vi "WindowArrayV0.42.vi"(0 "Searching center":dbl format="%.2f", 2 "X-axis":dbl[](array[numeric]) format="%.2f", 3 "The Data":dbl[](array[numeric]) format="%.2f", 5 "Window Width (point)":i32=80) -> (1 "scale":dbl format="%.2f", 4 "starting point":dbl format="%.2f", 6 "Closest peak position":dbl format="%.2f", 7 "X-Axis Subset":dbl[](array[numeric]) format="%.2f", 8 "Data Subset":dbl[](array[numeric]) format="%.2f")   [LabVIEW 2024]
doc: "Truncate the data around a peak. Normalize X-Axis so I can use the spline VI, and you can retrive the original X-Axis with *scale+StartingPoint."
uses:
  <vilib>/Analysis/NI_AALPro.lvlib
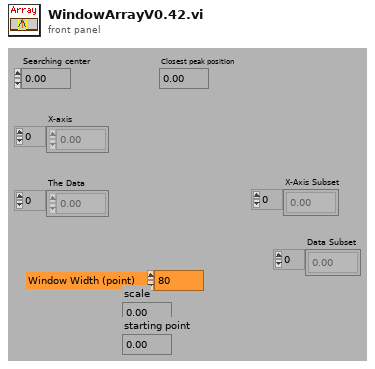
[diagram p1: front panel]
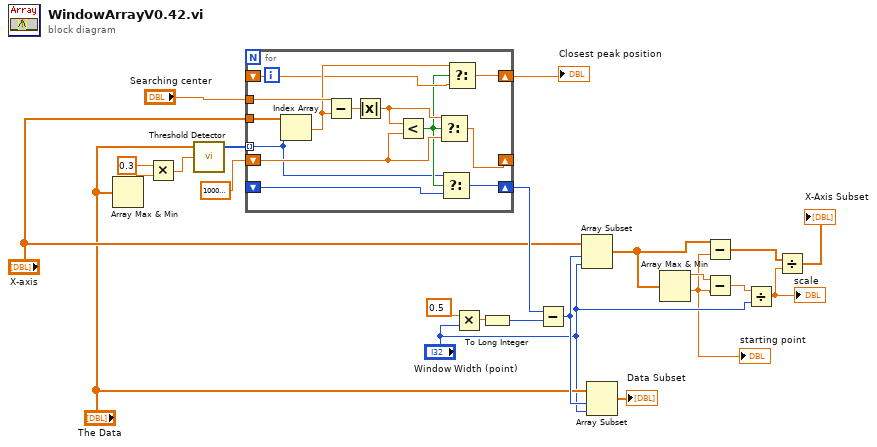
[diagram p0: block diagram]
diagram:
  n1 = Array Max & Min(array="The Data") -> (max value=w18:dbl)  [unwired: 3 out]
  n2 = Multiply(x=0.3, y=w18) -> (x*y=w20:dbl)
  n3 = call <vilib>:"Threshold Detector.vi"("threshold"=w20, "X"="The Data") -> ("Indices"=w17:i32[])  [unwired: 1 in, 2 out]
  n4 = for {
    tunnel: w17 -> [w25] mode=indexing
    tunnel: "X-axis" -> [w36]
    tunnel: "Searching center" -> [w35]
    shift-right: [w31] -> _
    shift-left: 1000000000.0 ("x") -> [w32]
    shift-right: [w29] -> w23
    shift-left: _ -> [w28]
    shift-right: [w26] -> w16
    shift-left: _ -> [w24]
    n5 = Index Array(array=w36, index=w25) -> (element=w30:dbl)
    n6 = Subtract(x=w35, y=w30) -> (x-y=w34:dbl)
    n7 = Absolute Value(x=w34) -> (abs(x)=w33:dbl)
    n8 = Less?(x=w33, y=w32) -> (x < y?=w27:bool)
    n9 = Select(t=w33, s=w27, f=w32) -> (s? t:f=w31:dbl)
    n10 = Select(t=w25, s=w27, f=w24) -> (s? t:f=w26:i32)
    n11 = Select(t=w30, s=w27, f=w28) -> (s? t:f=w29:dbl)
  }
  "Closest peak position" <- w23
  n12 = Multiply(x=sgl 0.5 ("y"), y="Window Width (point)") -> (x*y=w15:sgl)
  n13 = To Long Integer(number=w15) -> (32bit integer=w14:i32)
  n14 = Subtract(x=w16, y=w14) -> (x-y=w11:i32)
  n15 = Array Subset(array="X-axis", index=w11, length="Window Width (point)") -> (w4:dbl[])
  n16 = Array Subset(array="The Data", index=w11, length="Window Width (point)") -> (→"Data Subset":dbl[])
  n17 = Array Max & Min(array=w4) -> (max value=w8:dbl, min value=w5:dbl)  [unwired: 2 out]
  "starting point" <- w5
  n18 = Subtract(x=w4, y=w5) -> (x-y=w3:dbl[])
  n19 = Subtract(x=w8, y=w5) -> (x-y=w7:dbl)
  n20 = Divide(x=w7, y="Window Width (point)") -> (x/y=w2:dbl)
  "scale" <- w2
  n21 = Divide(x=w3, y=w2) -> (x/y=→"X-Axis Subset":dbl[])
